vi "Write Class Loader Enqueuer.vi"(8 "error in (no error)":errorcluster, 10 "Actor Framework:Message Enqueuer":refnum<class "Message Enqueuer.lvclass">, 11 "Test Caller Actor in":refnum<class "Test Caller Actor.lvclass">) -> (0 "error out":errorcluster, 3 "Test Caller Actor out":refnum<class "Test Caller Actor.lvclass">)   [LabVIEW 2023, in "Test Caller Actor.lvlib" / "Test Caller Actor.lvclass"]
uses:
  Test Caller Actor.lvclass
  Test Caller Actor.lvclass/Test Caller Actor.ctl
  <vilib>/ActorFramework/Message Enqueuer/Message Enqueuer.lvclass
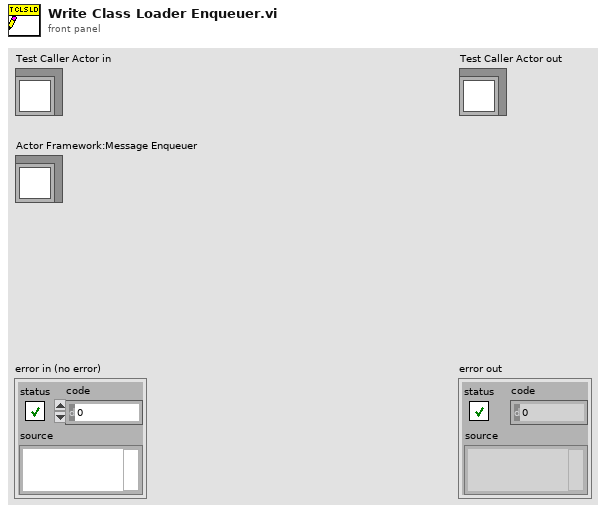
[diagram p1: front panel]
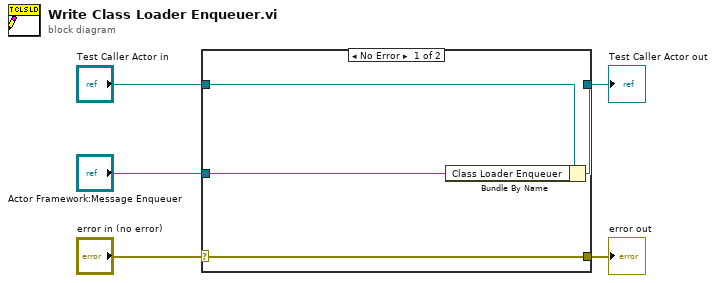
[diagram p0: block diagram]
diagram:
  n1 = case shown="No Error" "error in (no error)" {
    selector: "error in (no error)" -> [w9 w10]
    tunnel: [w9 w10] -> w4
    tunnel: [w7 w11] -> w2
    tunnel: "Test Caller Actor in" -> [w8 w11]
    tunnel: "Actor Framework:Message Enqueuer" -> [w6 _]
    frame No Error {
      n2 = Bundle By Name(cluster=w8, "Class Loader Enqueuer"=w6) -> (w7:refnum<class "Test Caller Actor.lvclass">)
    }
    frame Error {
    }
  }
  "error out" <- w4
  "Test Caller Actor out" <- w2
